vi "Log.vi"(8 "error in (no error)":errorcluster, 9 "Timestamp data points":bool, 10 "tdms file":refnum<k34>, 11 "Start Stream Result in":refnum<class "Start Stream Result.lvclass">) -> (0 "error out":errorcluster, 2 "tdms file out":refnum<k34>, 3 "Start Stream Result out":refnum<class "Start Stream Result.lvclass">)   [LabVIEW 2024, in "Start Stream Result.lvclass"]
uses:
  Start Stream Result.lvclass
  D:/GitHub/NHMFL_Core/Libraries/Instruments/Results/Acquired Result/Acquired Result.lvclass
  Start Stream Result.lvclass/Start Stream Result.ctl
  Acquired Result/Acquired Result.lvclass/Acquired Result.ctl
  Read dt.vi
  Read t0.vi
  Acquired Result/Read Group.vi
  Acquired Result/Read Channels.vi
  Read Scaling coefficients.vi
  Read Configuration.vi
  Acquired Result/Read Settings.vi
  Acquired Result/Acquired Result.lvclass
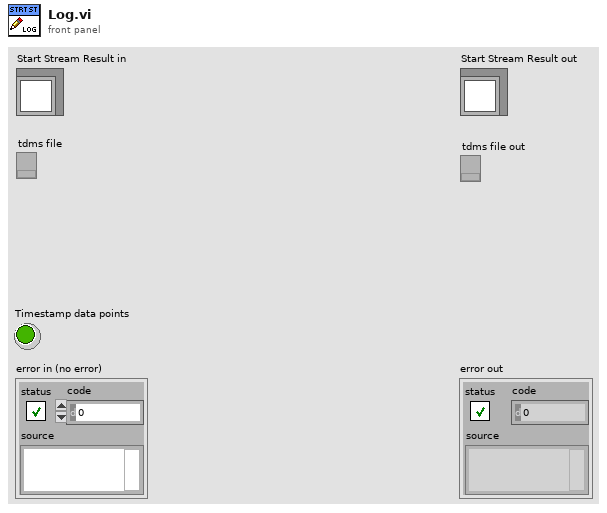
[diagram p1: front panel]
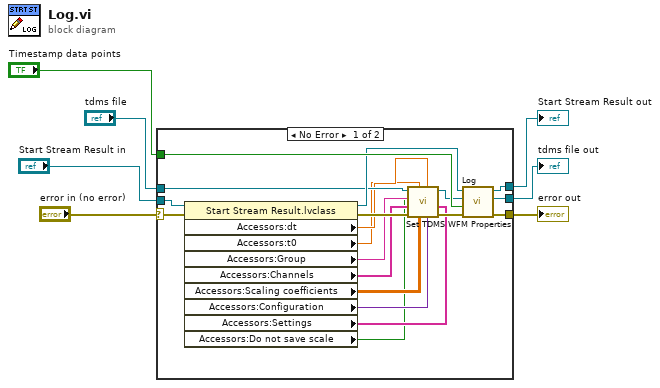
[diagram p0: block diagram]
diagram:
  n1 = case shown="No Error" "error in (no error)" {
    selector: "error in (no error)" -> [w11 w29]
    tunnel: [w26 w29] -> w7
    tunnel: [w25 w28] -> w6
    tunnel: [w24 w27] -> w5
    tunnel: "Timestamp data points" -> [w23 _]
    tunnel: "Start Stream Result in" -> [w20 w27]
    tunnel: "tdms file" -> [w17 w28]
    frame No Error {
      n2 = property class="Start Stream Result.lvclass"(reference=w20, error in=w11) -> (reference out=w19:refnum<class "Start Stream Result.lvclass">, error out=w21:errorcluster, "Accessors:dt"=w14:dbl, "Accessors:t0"=w13:dbl, "Accessors:Group"=w18:string, "Accessors:Channels"=w15:string[], "Accessors:Scaling coefficients"=w12:dbl[][], "Accessors:Configuration"=w10:variant, "Accessors:Settings"=w9:string[], "Accessors:Do not save scale"=w8:bool)
      n3 = call "Set TDMS WFM Properties.vi"("Settings"=w9, "Do not save scale"=w8, "Configuration"=w10, "dt"=w14, "Scaling coefficients"=w12, "t0"=w13, "error in (no error)"=w21, "Channel names"=w15, "Group name"=w18, "tdms file"=w17) -> ("error out"=w22:errorcluster, "tdms file out"=w16:refnum<k34>)
      n4 = call-parent "Log.vi"("error in (no error)"=w22, "Timestamp data points"=w23, "tdms file"=w16, "Acquired Result in"=w19) -> ("error out"=w26:errorcluster, "tdms file out"=w25:refnum<k34>, "Acquired Result out"=w24:refnum<class "Start Stream Result.lvclass">)  [unwired: 5 in]
    }
    frame Error {
    }
  }
  "error out" <- w7
  "Start Stream Result out" <- w5
  "tdms file out" <- w6
